vi "log_file_path.vi"(10 "base path in":path, 11 "base name in":string="SweepTable_") -> (2 "path out":path, 3 "string path out":string)   [LabVIEW 2012]
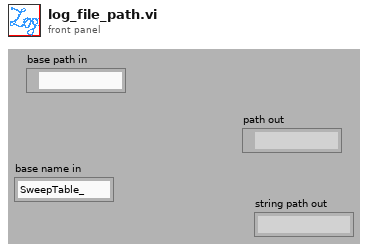
[diagram p1: front panel]
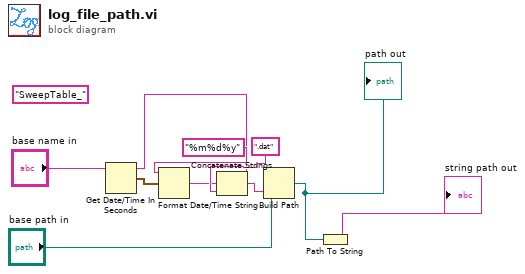
[diagram p0: block diagram]
diagram:
  (unwired) "SweepTable_" ("string")
  n1 = Get Date/Time In Seconds() -> (seconds since 1Jan1904=w9:timestamp)
  n2 = Format Date/Time String(time format string (%c)="%m%d%y", seconds (now)=w9) -> (date/time string=w6:string)  [unwired: 1 in]
  n3 = Concatenate Strings("base name in", w6, ".dat" ("string")) -> (w5:string)
  n4 = Build Path(base path="base path in", name or relative path=w5) -> (appended path=w3:path)
  "path out" <- w3
  n5 = Path To String(path=w3) -> (string=→"string path out":string)
